vi "DaQ_Signal_Deq.vi"(8 "Error In":errorcluster, 11 "Queue In":refnum<queue>) -> (0 "Error Out":errorcluster, 2 "Signal":waveform(dbl), 3 "Queue Out":refnum<queue>)   [LabVIEW 2021]
panel:
  # "Input"
  # "Output"
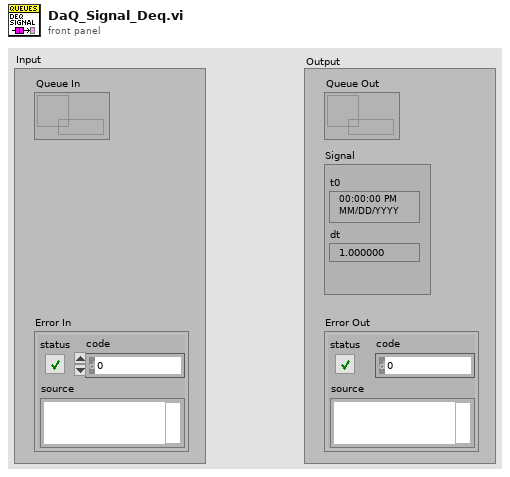
[diagram p1: front panel]
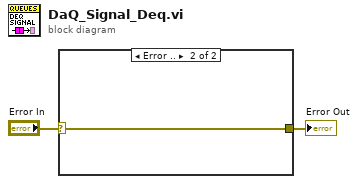
[diagram p0: block diagram]
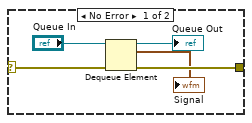
[diagram p2: hidden frame]
diagram:
  n1 = case shown="Error .." "Error In" {
    selector: "Error In" -> [w6 w8]
    tunnel: [w5 w8] -> w1
    frame No Error {
      n2 = Dequeue Element(queue="Queue In", error in (no error)=w6) -> (queue out=→"Queue Out":refnum<queue>, element=→"Signal":waveform(dbl), error out=w5:errorcluster)  [unwired: 1 in, 1 out]
    }
    frame Error {
    }
  }
  "Error Out" <- w1
